vi "auto spy shoot high.vi"(11 "High?":bool) -> ()   [LabVIEW 2015]
uses:
  <vilib>/Rock Robotics/WPI/Solenoid/WPI_SolenoidValue.ctl
  <vilib>/Rock Robotics/WPI/CAN/TalonSRX/WPI_CANTalonSRX_APIControlMode.ctl
  <vilib>/Rock Robotics/Network Tables/NT Read Number.vi
  <vilib>/Rock Robotics/WPI/Solenoid/WPI_SolenoidSetEnum.vi
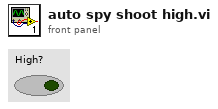
[diagram p1: front panel]
types:
  T1 = typedef "WPI_SolenoidDevRef.ctl" = cluster{"DevStatus":errorcluster, "Pneumatics Control Module":u8, "Forward Solenoid Channel":T2, "Reverse Solenoid Channel":T2}
  T2 = typedef "WPI_SolenoidChannel.ctl" = enum8{"Solenoid 0", "Solenoid 1", "Solenoid 2", "Solenoid 3", "Solenoid 4", "Solenoid 5", "Solenoid 6", "Solenoid 7", "Invalid"}
  T3 = typedef "WPI_MotorControlDeviceRef.ctl" = cluster{"DeviceStatus":errorcluster, "Type":T4, "PWM":cluster{"PWM Channel":T5, "DeadBand":T6}, "CAN":cluster{"Device Number":u8, "Control Mode":T7, "Semaphore":T8, "Max Vout":dbl, "TalonSRX Control Mode":T9}, "Invert":bool}
  T4 = typedef "WPI_MotorControlType.ctl" = enum16{"PWM", "CAN", "CANTalonSRX"}
  T5 = typedef "FPGA_DIOPWMChannel.ctl" = enum8{"PWM 0", "PWM 1", "PWM 2", "PWM 3", "PWM 4", "PWM 5", "PWM 6", "PWM 7", "PWM 8", "PWM 9", "PWM MXP 0", "PWM MXP 1", "PWM MXP 2", "PWM MXP 3", "PWM MXP 4", "PWM MXP 5", "PWM MXP 6", "PWM MXP 7", "PWM MXP 8", "PWM MXP 9", "Invalid"}
  T6 = typedef "WPI_PWMDeadband.ctl" = cluster{"Name":string, "maxPositivePwm":i32, "minPositivePwm":i32, "centerPwm":i32, "maxNegativePwm":i32, "minNegativePwm":i32, "angularRange":u16}
  T7 = typedef "WPI_CANJaguar_ControlMode.ctl" = enum8{"Percent VBus", "Current", "Speed", "Position", "Voltage"}
  T8 = typedef "Semaphore RefNum" = refnum<k1>
  T9 = typedef "WPI_CANTalonSRX_APIControlMode.ctl" = enum8{"Percent VBus", "Speed", "Position", "Slave", "Unchanged / Invalid", "Voltage Compensation", "Current", "Motion Profile"}
  T10 = typedef "WPI_SolenoidValue.ctl" = enum16{"Off", "On", "Forward", "Reverse"}
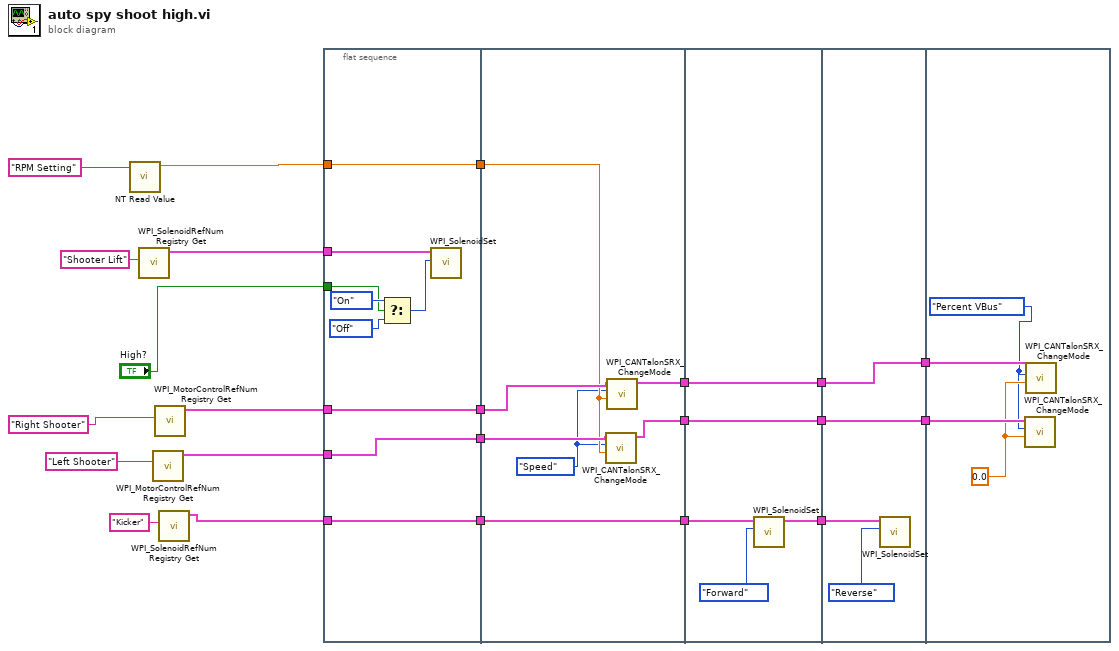
[diagram p0: block diagram]
diagram:
  n1 = call-poly <vilib>:"NT Read Value.vi"("Name"="RPM Setting") -> ("Numeric"=w15:dbl)  [unwired: 9 in, 1 out]
  n2 = call <vilib>:"WPI_SolenoidRefNum Registry Get.vi"("refnum name"="Shooter Lift") -> ("SolenoidDevRef"=w22:T1)  [unwired: 9 in, 1 out]
  n3 = call <vilib>:"WPI_MotorControlRefNum Registry Get.vi"("refnum name"="Left Shooter") -> ("MotorControlDevRef"=w17:T3)  [unwired: 9 in, 1 out]
  n4 = call <vilib>:"WPI_MotorControlRefNum Registry Get.vi"("refnum name"="Right Shooter") -> ("MotorControlDevRef"=w18:T3)  [unwired: 9 in, 1 out]
  n5 = call <vilib>:"WPI_SolenoidRefNum Registry Get.vi"("refnum name"="Kicker") -> ("SolenoidDevRef"=w12:T1)  [unwired: 9 in, 1 out]
  n6 = flat-sequence {
    tunnel: w22 -> [w32]
    tunnel: "High?" -> [w28]
    tunnel: [w27] -> w19
    tunnel: w18 -> [w27]
    tunnel: w17 -> [w26]
    tunnel: [w26] -> w16
    tunnel: w15 -> [w25]
    tunnel: [w25] -> w14
    tunnel: w12 -> [w24]
    tunnel: [w24] -> w11
    tunnel: w19 -> [w39]
    tunnel: w16 -> [w38]
    tunnel: w14 -> [w37]
    tunnel: w11 -> [w36]
    tunnel: [w36] -> w10
    tunnel: [w35] -> w8
    tunnel: [w34] -> w3
    tunnel: w10 -> [w44]
    tunnel: [w42] -> w9
    tunnel: w8 -> [w41]
    tunnel: [w41] -> w7
    tunnel: [w40] -> w4
    tunnel: w3 -> [w40]
    tunnel: w9 -> [w48]
    tunnel: w7 -> [w46]
    tunnel: [w46] -> w6
    tunnel: [w45] -> w5
    tunnel: w4 -> [w45]
    tunnel: w6 -> [w52]
    tunnel: w5 -> [w51]
    frame #0 {
      n7 = Select(t=WPI_SolenoidValue."On" ("Value"), s=w28, f=WPI_SolenoidValue."Off" ("Value")) -> (s? t:f=w29:T10)
      n8 = call-poly <vilib>:"WPI_SolenoidSet.vi"("Value"=w29, "SolenoidDevRef"=w32) -> ()  [unwired: 8 in, 2 out]
    }
    frame #1 {
      w33 = WPI_CANTalonSRX_APIControlMode."Speed" ("Control Mode")
      n9 = call <vilib>:"WPI_CANTalonSRX_ChangeMode.vi"("Output"=w37, "Control Mode"=w33, "CAN Talon SRX Ref"=w38) -> ("CAN Talon SRX Ref"=w34:T3)  [unwired: 7 in, 1 out]
      n10 = call <vilib>:"WPI_CANTalonSRX_ChangeMode.vi"("Output"=w37, "Control Mode"=w33, "CAN Talon SRX Ref"=w39) -> ("CAN Talon SRX Ref"=w35:T3)  [unwired: 7 in, 1 out]
    }
    frame #2 {
      n11 = call-poly <vilib>:"WPI_SolenoidSet.vi"("Value"=WPI_SolenoidValue."Forward", "SolenoidDevRef"=w44) -> ("SolenoidDevRef"=w42:T1)  [unwired: 8 in, 1 out]
    }
    frame #3 {
      n12 = call-poly <vilib>:"WPI_SolenoidSet.vi"("Value"=WPI_SolenoidValue."Reverse", "SolenoidDevRef"=w48) -> ()  [unwired: 8 in, 2 out]
    }
    frame #4 {
      w49 = WPI_CANTalonSRX_APIControlMode."Percent VBus" ("Control Mode")
      w50 = 0.0 ("Output")
      n13 = call <vilib>:"WPI_CANTalonSRX_ChangeMode.vi"("Output"=w50, "Control Mode"=w49, "CAN Talon SRX Ref"=w51) -> ()  [unwired: 7 in, 2 out]
      n14 = call <vilib>:"WPI_CANTalonSRX_ChangeMode.vi"("Output"=w50, "Control Mode"=w49, "CAN Talon SRX Ref"=w52) -> ()  [unwired: 7 in, 2 out]
    }
  }
